vi "CPP_VeerSpectra.vi"() -> (5 "Plug in titles":string[](array[string]), 7 "Plug in values":string[](array[string]))   [LabVIEW 2011]
uses:
  Controls/Instrument_Array.ctl
  Controls/Post_Process.ctl
  Controls/Graph_Type.ctl
  Globals/Meas_global.vi
  Acquisition/PWA/PWAtasksGLOBAL.vi
  Globals/Plug_in_data_global.vi
panel:
  out "dF/ Hz":dbl
  in  "Inst Array":T1=enum."Analogue"
  in  "Show Smooth":bool=TRUE
  in  "Save Spectra?":bool
  in  "Desired number of samples per block":i32=32768
  in  "Calculate Spectra and Histogram?":bool=TRUE
  out "Spectra":cluster{dbl, dbl, "Spectrum output array":dbl[]}(graph)
  in  "Averaging samples":i32=1 min=1 max=1000
  in  "Spectra Index (from ALL channels)":i32
  out "Waveform Graph":dbl[][](graph)
  in  "Channels to Plot":i32[](array[ring])=[0, 1, 2, 3] items=["RV (Mic1)", "RV (Mic2)", "RV (Mic3)", "RV (Mic4)", "Save Nothing"]
  # "Run this VI to update the channel names"
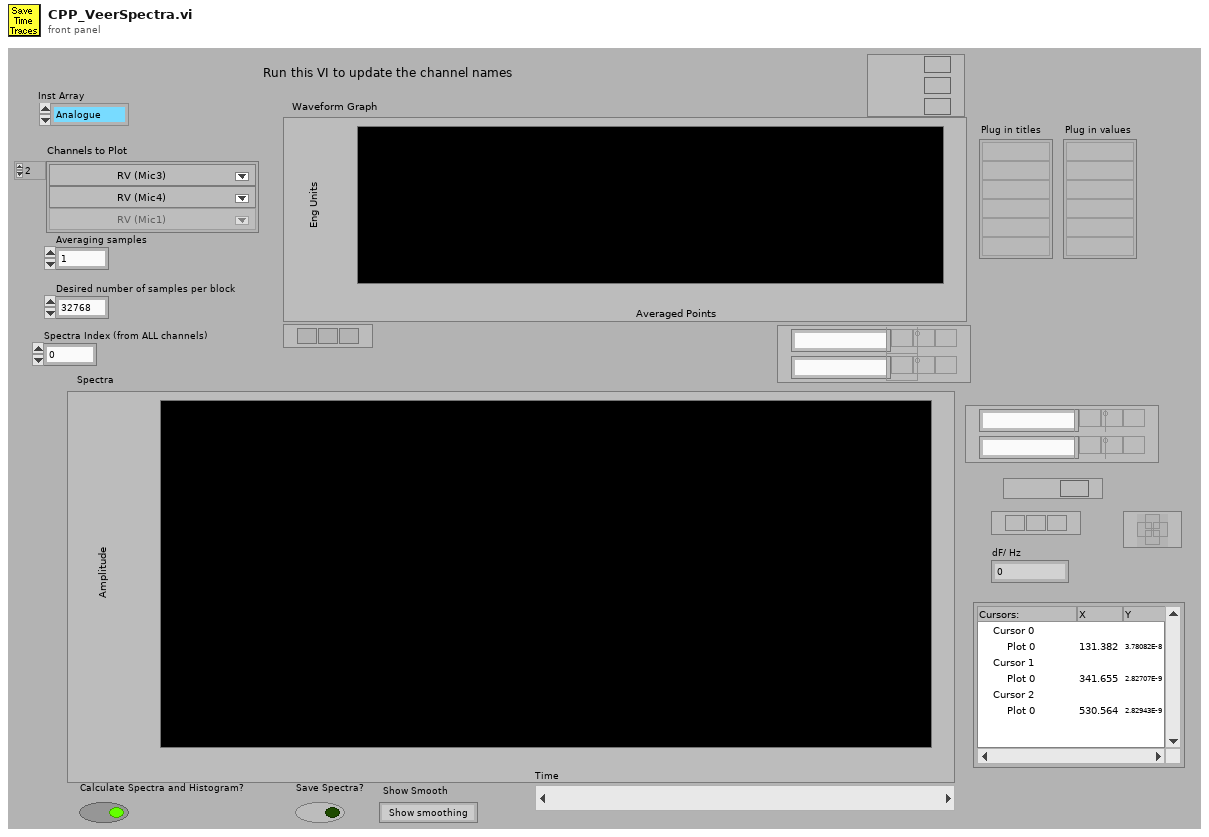
[diagram p1: front panel]
types:
  T1 = typedef "Instrument_Array.ctl" = enum16{"PWA", "LDA", "Analogue"}
  T2 = typedef "Analysis_info_cluster.ctl" = cluster{"Colour":u32, "Inst type":T3, "Inst name":string, "Symbol":string, "Code name":string, "Extra Info":string, "Inst Array":T1, "Index":i32, "Voltage Index":i32, "Extra Titles":string[], "Extra Values":string[]}
  T3 = typedef "Inst_type.ctl" = enum16{"Propeller anemometer", "Raw voltage", "Pressure Transducer", "Pitot-static tube", "Preston tube", "Hot wire", "Cross wire 1", "Cross wire 2", "Generic Linear", "Generic Polynomial", "Generic BackPoly", "Fast FID", "Thermocouple", "Cold wire", "Pulsed Wire", "LDA Vel", "LDA Tran time", "LDA Arr time"}
  T4 = typedef "Post_Process.ctl" = enum16{"Take New Data", "Post Process Raw Data File"}
  T5 = typedef "Graph_Type.ctl" = enum16{"Show no graph", "Voltage trace", "Velocity trace", "Vel histogram", "Spectrum", "f.E(f) v Log f", "Auto-Corr"}
  T6 = cluster{"Plot 1":u16, "Plot 2":u16, "Save graph":u16, "Plot Type":T5}
  T7 = cluster{dbl, dbl, "Spectrum output array":dbl[]}[]
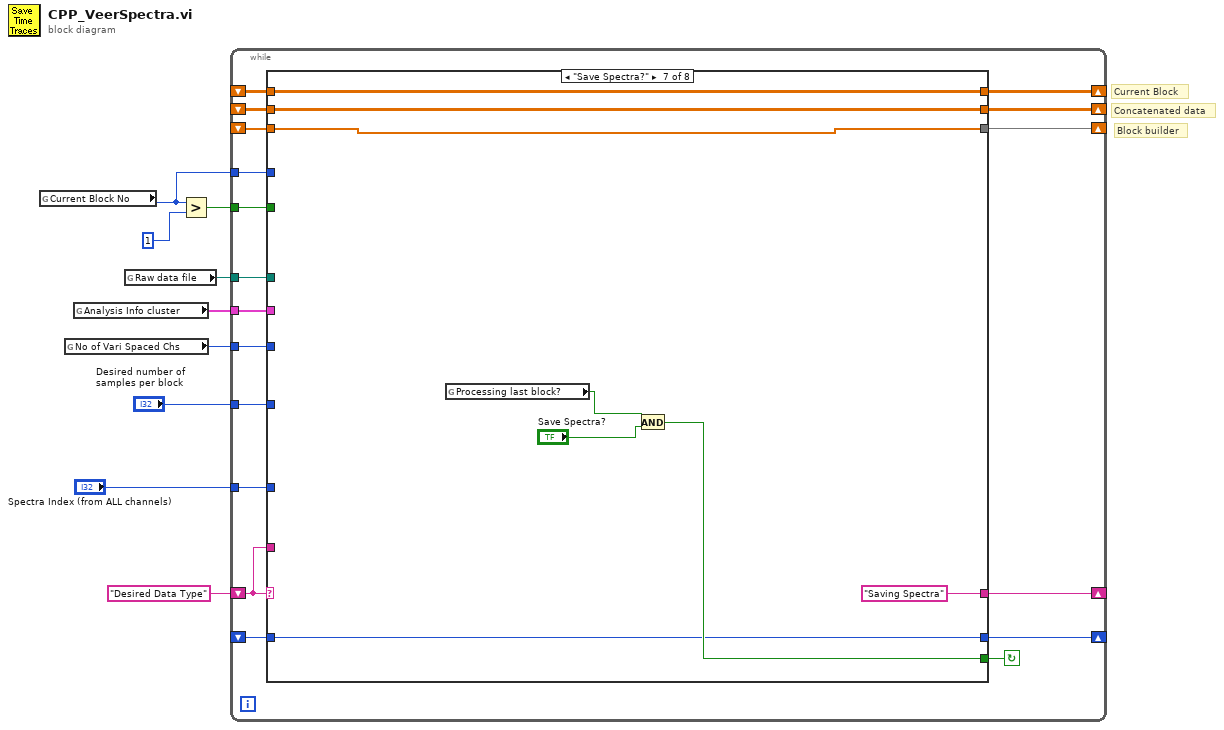
[diagram p0: block diagram]
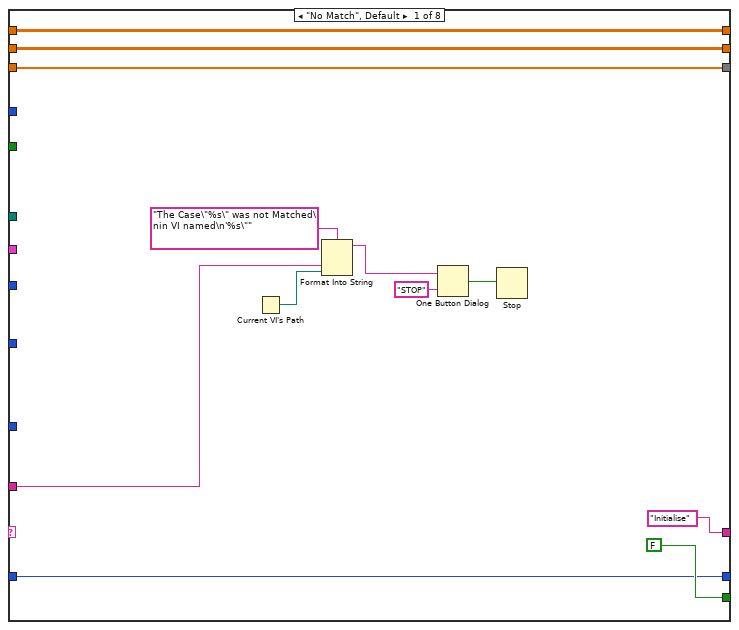
[diagram p2: hidden frame]
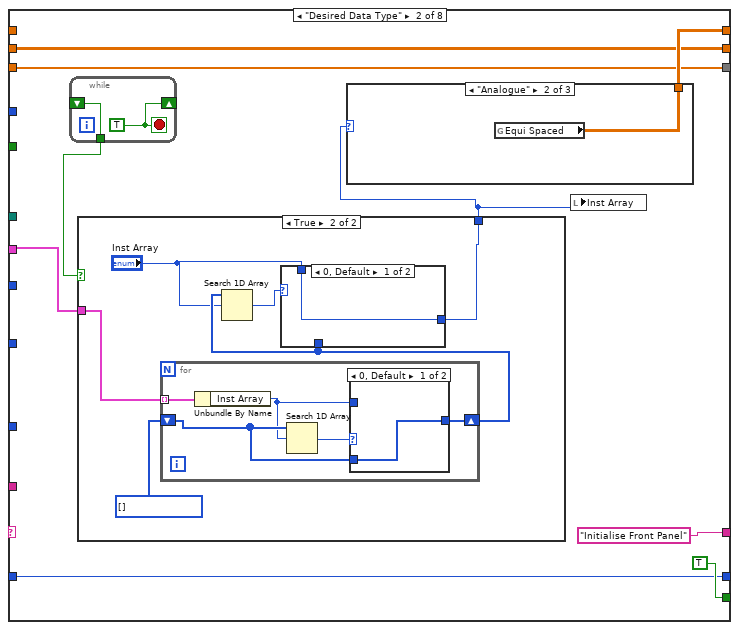
[diagram p3: hidden frame]
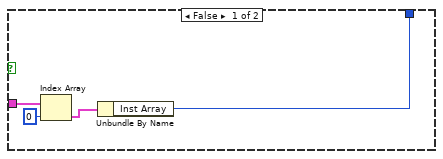
[diagram p4: hidden frame]
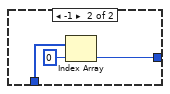
[diagram p5: hidden frame]
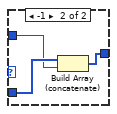
[diagram p6: hidden frame]
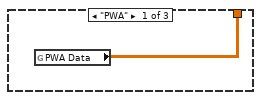
[diagram p7: hidden frame]
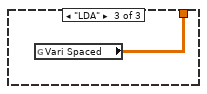
[diagram p8: hidden frame]
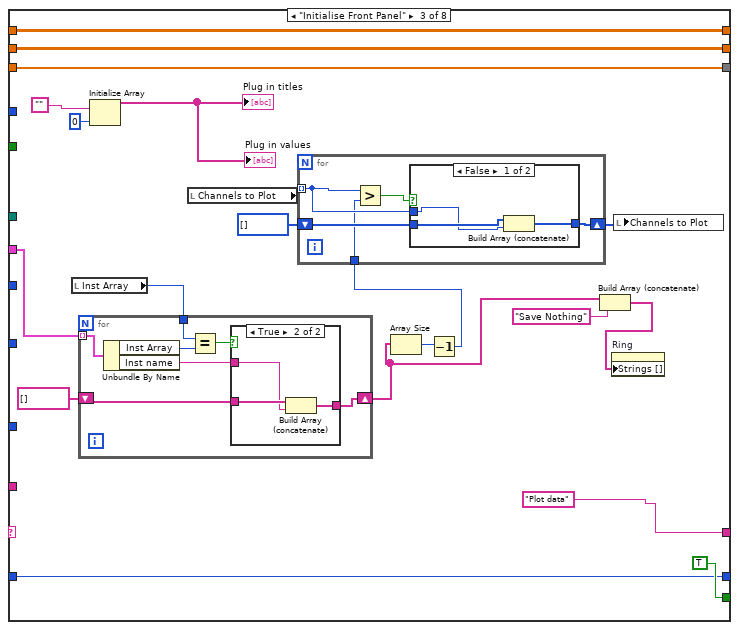
[diagram p9: hidden frame]
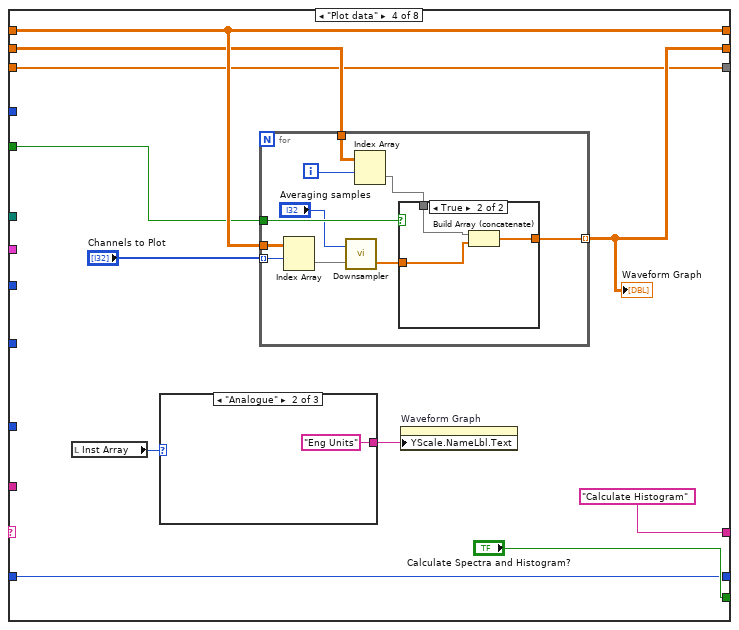
[diagram p12: hidden frame]
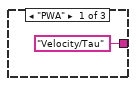
[diagram p13: hidden frame]
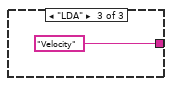
[diagram p14: hidden frame]
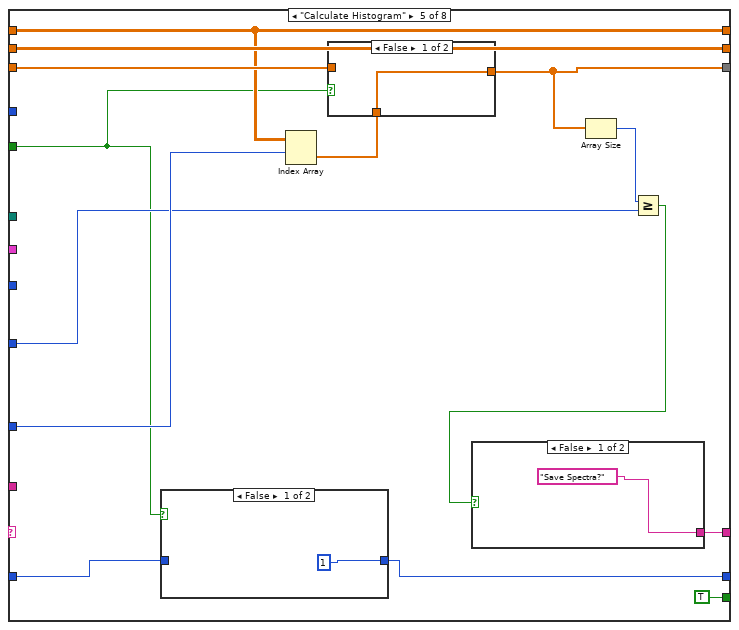
[diagram p16: hidden frame]
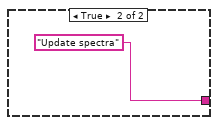
[diagram p18: hidden frame]
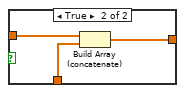
[diagram p19: hidden frame]
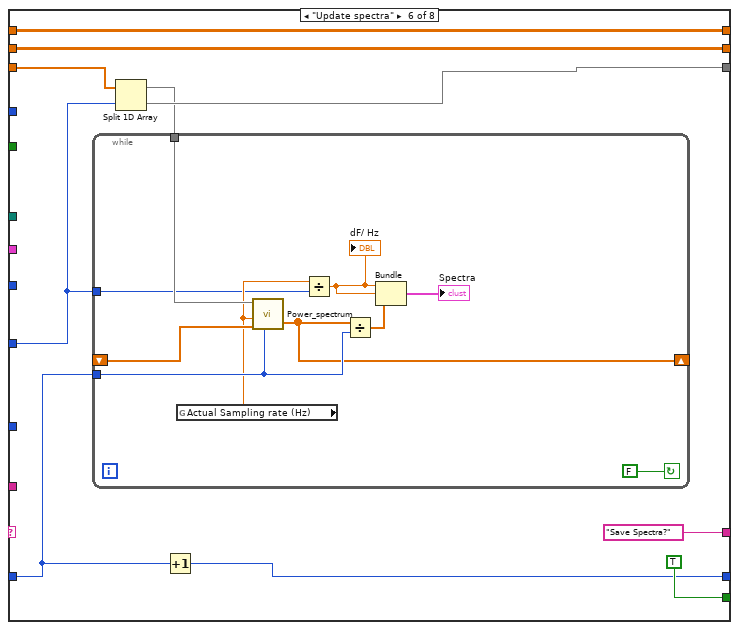
[diagram p20: hidden frame]
diagram:
  # "Block builder"
  # "Concatenated data"
  # "Current Block"
  n1 = global read "Meas_global.vi" "Current Block No"() -> (w6:i32)
  n2 = global read "Meas_global.vi" "No of Vari Spaced Chs"() -> (w4:i32)
  n3 = global read "Meas_global.vi" "Analysis Info cluster"() -> (w5:T2[])
  n4 = global read "Meas_global.vi" "Raw data file"() -> (w8:path)
  n5 = Greater?(x=w6, y=1) -> (0:w3:bool)
  n6 = while {
    shift-left: "Desired Data Type" -> [w25]
    shift-right: [w26] -> _
    tunnel: w8 -> [w24]
    tunnel: w3 -> [w23]
    tunnel: w6 -> [w22]
    tunnel: w5 -> [w21]
    tunnel: w4 -> [w20]
    shift-right: [w19] -> _
    shift-left: _ -> [w18]
    shift-right: [w16] -> _
    shift-left: _ -> [w17]
    shift-right: [w14] -> _
    shift-left: _ -> [w15]
    tunnel: "Desired number of samples per block" -> [w13]
    tunnel: "Spectra Index (from ALL channels)" -> [w12]
    shift-right: [w11] -> _
    shift-left: _ -> [w10]
    stop <- w27 continue-if-true
    n7 = case shown="\"Save Spectra?\"" w25 {
      tunnel: [FALSE TRUE TRUE "Calculate Spectra and Histogram?" TRUE ("Calculate Spectra and Histogram?") TRUE ("Calculate Spectra and Histogram?") w188 FALSE ("Calculate Spectra and Histogram?")] -> w27
      tunnel: ["Initialise" "Initialise Front Panel" "Plot data" "Calculate Histogram" ("t") w148 "Save Spectra?" "Saving Spectra" w201] -> w26
      tunnel: w25 -> [w34 _ _ _ _ _ _ _]
      tunnel: w24 -> [_ _ _ _ _ _ _ _]
      tunnel: w23 -> [_ _ _ w125 w147 _ _ _]
      tunnel: w22 -> [_ _ _ _ _ _ _ _]
      tunnel: w21 -> [_ w41 w80 _ _ _ _ w199]
      tunnel: w20 -> [_ _ _ _ _ _ _ _]
      tunnel: [w31 w46 w86 w127 w156 w175 w193 w202] -> w19
      tunnel: w18 -> [w31 _ w86 w127 w156 w175 w193 w202]
      tunnel: w17 -> [w30 w45 w85 w126 w157 w176 w194 w203]
      tunnel: [w30 w45 w85 w123 w157 w176 w194 w203] -> w16
      tunnel: w15 -> [w29 w44 w82 w120 w158 w174 w191 w200]
      tunnel: [w29 w44 w82 w120 w154 w173 w191 w200] -> w14
      tunnel: w13 -> [_ _ _ _ w150 w169 _ w196]
      tunnel: w12 -> [_ _ _ _ w152 _ _ w198]
      tunnel: [w28 w43 w81 w119 w146 w167 w187 w195] -> w11
      tunnel: w10 -> [w28 w43 w81 w119 w145 w168 w187 w195]
      frame "No Match", Default {
        n8 = Current VI's Path() -> (path=w33:path)
        n9 = Format Into String(format string="The Case\"%s\" was not Matched\nin VI named\n'%s\"" ("Format String"), w34, w33) -> (resulting string=w37:string)  [unwired: 2 in, 1 out]
        n10 = One Button Dialog(message=w37, button name ("OK")="STOP") -> (true=w35:bool)
        n11 = Stop(stop? (T)=w35) -> ()
      }
      frame "Desired Data Type" {
        n12 = while {
          shift-right: [w73] -> _
          shift-left: _ -> [w72]
          tunnel: [w72] -> w42
          stop <- w73 stop-if-true
          w73 = TRUE
        }
        n13 = case shown="True" w42 {
          tunnel: w41 -> [w52 w58]
          tunnel: [w49 w54] -> w40
          frame False {
            n14 = Index Array(array=w52, index=0) -> (element=w50:T2)
            n15 = Unbundle By Name(w50) -> ("Inst Array"=w49:T1)
          }
          frame True {
            w57 = T1[] [] items=["PWA", "LDA", "Analogue"]
            n16 = for {
              tunnel: w58 -> [w67] mode=indexing
              shift-right: [w63] -> w55
              shift-left: w57 -> [w65]
              n17 = Unbundle By Name(w67) -> ("Inst Array"=w64:T1)
              n18 = Search 1D Array(1D array=w65, element=w64) -> (index of element=w66:i32)  [unwired: 1 out]
              n19 = case shown="0, Default" w66 {
                tunnel: w65 -> [w68 w71]
                tunnel: w64 -> [_ w70]
                tunnel: [w68 w69] -> w63
                frame 0, Default {
                }
                frame -1 {
                  n20 = Build Array (concatenate)(w71, w70) -> (w69:T1[])
                }
              }
            }
            n21 = Search 1D Array(1D array=w55, element="Inst Array") -> (index of element=w56:i32)  [unwired: 1 out]
            n22 = case shown="0, Default" w56 {
              tunnel: w55 -> [_ w61]
              tunnel: [w59 w60] -> w54
              tunnel: "Inst Array" -> [w59 _]
              frame 0, Default {
              }
              frame -1 {
                n23 = Index Array(array=w61, index=0) -> (element=w60:T1)
              }
            }
          }
        }
        n24 = case shown="\"Analogue\"" w40 {
          tunnel: [w74 w75 w76] -> w46
          frame "PWA" {
            n25 = global read "PWAtasksGLOBAL.vi" "PWA Data"() -> (w74:dbl[][])
          }
          frame "Analogue" {
            n26 = global read "Plug_in_data_global.vi" "Equi Spaced"() -> (w75:dbl[][])
          }
          frame "LDA" {
            n27 = global read "Plug_in_data_global.vi" "Vari Spaced"() -> (w76:dbl[][])
          }
        }
        n28 = local write "Inst Array"(w40) -> ()
      }
      frame "Initialise Front Panel" {
        n29 = local read "Inst Array"() -> (w79:T1)
        n30 = for {
          tunnel: w79 -> [w102]
          tunnel: w80 -> [w101] mode=indexing
          shift-right: [w98] -> w78
          shift-left: string[] [] -> [w99]
          n31 = Unbundle By Name(w101) -> ("Inst Array"=w103:T1, "Inst name"=w97:string)
          n32 = Equal?(x=w102, y=w103) -> (x = y?=w100:bool)
          n33 = case shown="True" w100 {
            tunnel: w99 -> [w104 w107]
            tunnel: [w104 w106] -> w98
            tunnel: w97 -> [_ w105]
            frame False {
            }
            frame True {
              n34 = Build Array (concatenate)(w107, w105) -> (w106:string[])
            }
          }
        }
        n35 = Initialize Array("", 0) -> (→"Plug in values" →"Plug in titles":string[])
        n36 = local read "Channels to Plot"() -> (w93:i32[])
        n37 = Array Size(array=w78) -> (size(s)=w88:i32)
        n38 = Decrement(x=w88) -> (x-1=w87:i32)
        n39 = for {
          tunnel: w93 -> [w109] mode=indexing
          shift-right: [w110] -> w91
          shift-left: i32[] [] -> [w111]
          tunnel: w87 -> [w108]
          n40 = Greater?(x=w109, y=w108) -> (0:w112:bool)
          n41 = case shown="False" w112 {
            tunnel: w111 -> [w115 w116]
            tunnel: [w114 w116] -> w110
            tunnel: w109 -> [w113 _]
            frame False {
              n42 = Build Array (concatenate)(w115, w113) -> (w114:i32[])
            }
            frame True {
            }
          }
        }
        n43 = Build Array (concatenate)(w78, "Save Nothing") -> (w89:string[])
        n44 = property on="Ring" class="Ring (strict)"("Strings []"=w89) -> ()  [unwired: 2 in, 2 out]
        n45 = local write "Channels to Plot"(w91) -> ()
      }
      frame "Plot data" {
        n46 = local read "Inst Array"() -> (w118:T1)
        n47 = case shown="\"Analogue\"" w118 {
          tunnel: ["Velocity/Tau" "Eng Units" "Velocity"] -> w117
          frame "PWA" {
          }
          frame "Analogue" {
          }
          frame "LDA" {
          }
        }
        n48 = for {
          tunnel: w127 -> [w140]
          tunnel: "Channels to Plot" -> [w139] mode=indexing
          tunnel: w126 -> [w136]
          tunnel: [w137] -> w123 mode=indexing
          tunnel: w125 -> [w138]
          i -> [w135]
          n49 = Index Array(array=w140, index (row)=w139) -> (element=w133:dbl[])  [unwired: 1 in]
          n50 = call "Downsampler.vi"("Input Array"=w133, "Averaging samples"="Averaging samples") -> ("Downsampled Array"=w132:dbl[])  [unwired: 1 out]
          n51 = Index Array(array=w136, index (row)=w135) -> (element=w134:dbl[])  [unwired: 1 in]
          n52 = case shown="True" w138 {
            tunnel: w134 -> [_ w144]
            tunnel: w132 -> [w141 w143]
            tunnel: [w141 w142] -> w137
            frame False {
            }
            frame True {
              n53 = Build Array (concatenate)(w144, w143) -> (w142:dbl[])
            }
          }
        }
        "Waveform Graph" <- w123
        n54 = property on="Waveform Graph" class="WFGraph (strict)"("YScale.NameLbl.Text"=w117) -> ()  [unwired: 2 in, 2 out]
      }
      frame "Calculate Histogram" {
        n55 = case shown="False" w147 {
          tunnel: [1 w160] -> w146
          tunnel: w145 -> [_ w160]
          frame False {
          }
          frame True {
          }
        }
        n56 = Index Array(array=w156, index (row)=w152) -> (element=w155:dbl[])  [unwired: 1 in]
        n57 = case shown="False" w147 {
          tunnel: w158 -> [_ w166]
          tunnel: [w163 w165] -> w154
          tunnel: w155 -> [w163 w164]
          frame False {
          }
          frame True {
            n58 = Build Array (concatenate)(w166, w164) -> (w165:dbl[])
          }
        }
        n59 = Array Size(array=w154) -> (size(s)=w153:i32)
        n60 = Greater Or Equal?(x=w153, y=w150) -> (x >= y?=w149:bool)
        n61 = case shown="False" w149 {
          tunnel: ["Save Spectra?" ("f") "Update spectra"] -> w148
          frame False {
          }
          frame True {
          }
        }
      }
      frame "Update spectra" {
        n62 = Split 1D Array(array=w174, index=w169) -> (first subarray=w170:dbl[], second subarray=w173:dbl[])
        n63 = while {
          shift-left: _ -> [w184]
          shift-right: [w177] -> _
          tunnel: w170 -> [w185]
          tunnel: w168 -> [w183]
          tunnel: w169 -> [w181]
          stop <- FALSE continue-if-true
          n64 = global read "Meas_global.vi" "Actual Sampling rate (Hz)"() -> (w182:dbl)
          n65 = call "Power_spectrum.vi"("U"=w185, "Sampling frequency"=w182, "Spectrum input array"=w184, "Block No"=w183) -> ("Spectrum output array"=w177:dbl[])  [unwired: 1 in, 1 out]
          n66 = Divide(x=w182, y=w181) -> (x/y=w179:dbl)
          "dF/ Hz" <- w179
          n67 = Divide(x=w177, y=w183) -> (x/y=w178:dbl[])
          n68 = Bundle(w179, w179, w178) -> (→"Spectra":cluster{dbl, dbl, dbl[]})  [unwired: 1 out]
        }
        n69 = Increment(x=w168) -> (x+1=w167:i32)
      }
      frame "Save Spectra?" {
        n70 = global read "Meas_global.vi" "Processing last block?"() -> (w189:bool)
        n71 = And(x=w189, y="Save Spectra?") -> (x .and. y?=w188:bool)
      }
      frame "Saving Spectra" {
        n72 = stacked-sequence {
          seq-local: [w207 _ _ _] -> [_ _ w240 _]
          seq-local: [_ w227 _ _] -> [_ _ w239 _]
          tunnel: [_ _ "Save Spectra?" _] -> w201
          tunnel: w199 -> [_ _ w246 _]
          tunnel: w198 -> [_ _ w245 _]
          tunnel: w196 -> [w205 _ _ _]
          tunnel: w195 -> [_ w225 _ _]
          frame #0 {
            n73 = global read "Meas_global.vi" "Post Process"() -> (w209:T4)
            n74 = Equal?(x=w209, y=Post_Process."Take New Data" ("Post Process")) -> (x = y?=w210:bool)
            n75 = case shown="False" w210 {
              tunnel: [w218 w222] -> w211
              frame False {
                n76 = global read "Meas_global.vi" "Pre Setup String"() -> (w219:string)
                n77 = call "Get_value_from_string.vi"("Input string"=w219, "Variable name"="Seconds since 1/1/04") -> ("Value"=w218:dbl)  [unwired: 1 in, 1 out]
              }
              frame True {
                n78 = Get Date/Time In Seconds() -> (seconds since 1Jan1904=w221:timestamp)
                n79 = To Double Precision Float(number=w221) -> (double precision float=w222:dbl)
              }
            }
            n80 = To Unsigned Long Integer(number=w211) -> (unsigned 32bit integer=w215:u32)
            n81 = Get Date/Time String(date format (0)=enum16{"short", "long", "abbreviated"}."abbreviated", seconds (now)=w215) -> (date string=w213:string, time string=w214:string)  [unwired: 1 out]
            n82 = Number To Decimal String(number=w215) -> (decimal integer string=w216:string)  [unwired: 1 out]
            n83 = Number To Decimal String(number=w205) -> (decimal integer string=w204:string)  [unwired: 1 out]
            n84 = Build Array("Time of meas", w213, w214, w216, "Block Length" ("element"), w204) -> (w207:string[])
          }
          frame #1 {
            n85 = global read "Meas_global.vi" "Actual Sampling rate (Hz)"() -> (w228:dbl)
            n86 = Decrement(x=w225) -> (x-1=w224:i32)
            n87 = global read "Meas_global.vi" "Raw data file"() -> (w234:path)
            n88 = global read "Meas_global.vi" "Comments"() -> (w233:string)
            n89 = Number To Decimal String(number=w224) -> (decimal integer string=w223:string)  [unwired: 1 out]
            n90 = Number To Fractional String(number=w228, precision (6)=i16 2) -> (F-format string=w231:string)  [unwired: 2 out]
            n91 = call "Path_2_String.vi"("Real Path"=w234) -> ("Path String"=w235:string)
            n92 = Build Array("No of Blocks", w223, "Frequency (Hz)", w231, "Raw Data file", w235, w233) -> (w227:string[])
          }
          frame #2 {
            n93 = Index Array(array=w246, index=w245) -> (element=w244:T2)
            n94 = Unbundle By Name(w244) -> ("Inst name"=w243:string)
            n95 = Build Array (concatenate)(w240, w239) -> (w238:string[])
            n96 = Build Array(w243) -> (w242:string[])
            n97 = local read "Spectra"() -> (w249:cluster{dbl, dbl, "Spectrum output array":dbl[]})
            n98 = Build Array(w238) -> (w237:string[][])
            n99 = Build Array(w249) -> (w248:T7)
            n100 = call "Plot_to_file.vi"("Show Smooth"="Show Smooth", "Start trace No"=0, "Trace names"=w242, "Graph"=T6 {"Plot 1"=1, "Plot 2"=0, "Save graph"=1, "Plot Type"=enum."Spectrum"}, "Plot file label"=w237, "Plot data"=w248) -> ()  [unwired: 6 out]
          }
          frame #3 {
            n101 = local write "Show Smooth"(FALSE ("Show Smooth")) -> ()
          }
        }
      }
    }
  }
